vi "Base_eleve.vi"() -> ()   [LabVIEW 2018]
uses:
  <vilib>/Instr/_visa.llb/VISA Configure Serial Port (Instr).vi
panel:
  out "Array 3":dbl[](array[numeric])
  out "Array 2":dbl[](array[numeric])
  out "Array":dbl[](array[numeric])
  out "Humidity":dbl[](graph)
  out "Pressure":dbl[](graph)
  out "Temperature":dbl[](graph)
  out "Humidity":dbl
  out "Pressure":dbl
  out "Temperature":dbl
  out "Chaîne":string
  in  "stop":bool
  in  "Nom de ressource VISA":refnum<visa-resource-name>
  # "1. Brancher la carte Arduino sur un port USB\n2. Choisir le port COM de la carte dans la liste déroulante \"Nom de ressource VISA\"\n3. Lancer le programme"
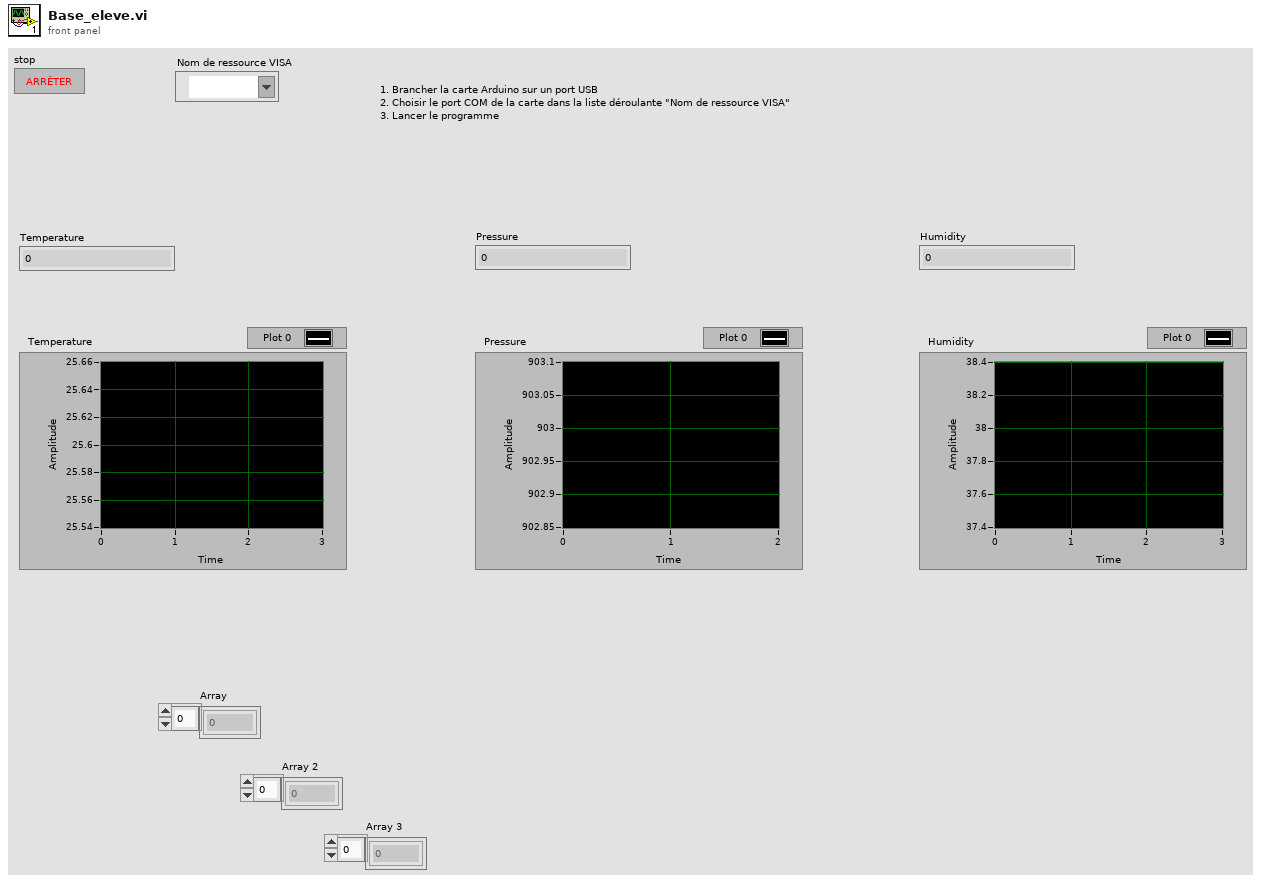
[diagram p1: front panel]
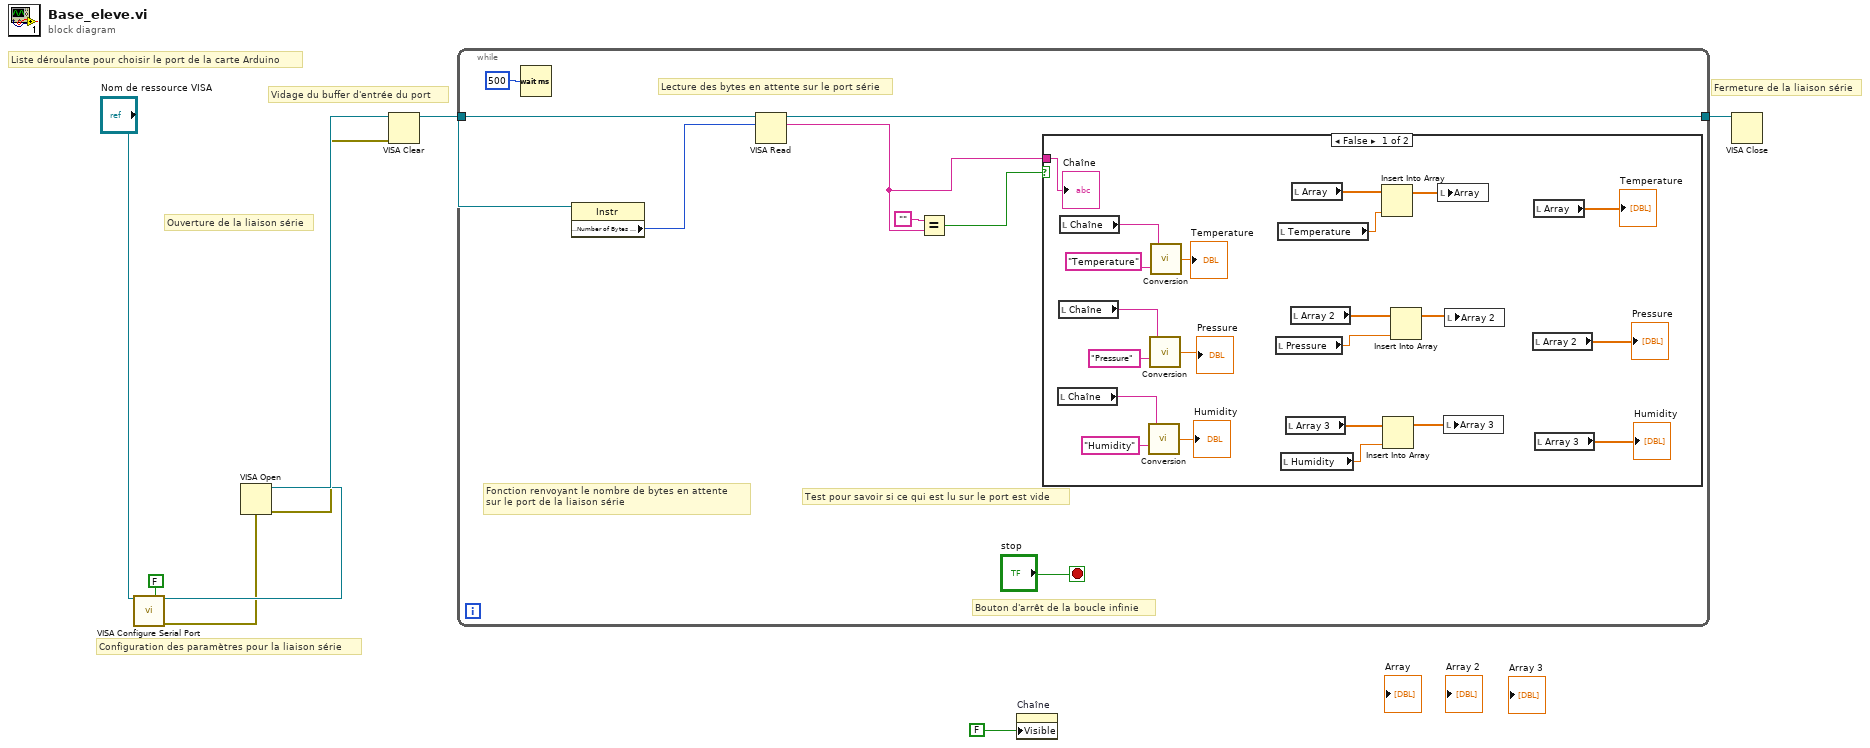
[diagram p0: block diagram]
diagram:
  # "Vidage du buffer d'entrée du port"
  # "Ouverture de la liaison série"
  # "Configuration des paramètres pour la liaison série"
  # "Liste déroulante pour choisir le port de la carte Arduino"
  # "Fermeture de la liaison série"
  n1 = call-poly "VISA Configure Serial Port"("VISA resource name"="Nom de ressource VISA", "Enable Termination\nChar (T)"=FALSE ("Enable Termination\nChar (T)")) -> ("VISA resource name out"=w6:refnum<visa-resource-name>, "error out"=w4:errorcluster)  [unwired: 12 in]
  n2 = VISA Open(error in (no error)=w4, VISA resource name=w6) -> (VISA resource name=w8:refnum<visa-resource-name>, error out=w3:errorcluster)  [unwired: 3 in]
  n3 = VISA Clear(VISA resource name=w8, error in (no error)=w3) -> (VISA resource name out=w7:refnum<visa-resource-name>)  [unwired: 1 out]
  n4 = while {
    tunnel: w7 -> [w16]
    tunnel: [w14] -> w2
    stop <- "stop" stop-if-true
    # "Lecture des bytes en attente sur le port série"
    # "Fonction renvoyant le nombre de bytes en attente\nsur le port de la liaison série"
    # "Test pour savoir si ce qui est lu sur le port est vide"
    # "Bouton d'arrêt de la boucle infinie"
    n5 = Wait (ms)(milliseconds to wait=u32 500 ("attente (ms)")) -> ()  [unwired: 1 out]
    n6 = property class="Instr"(reference=w16) -> ("Serial Settings:Number of Bytes at Serial Port"=w15:u32)  [unwired: 1 in, 2 out]
    n7 = VISA Read(VISA resource name=w16, byte count=w15) -> (VISA resource name out=w14:refnum<visa-resource-name>, read buffer=w10:string)  [unwired: 1 in, 2 out]
    n8 = Equal?(x="", y=w10) -> (x = y?=w11:bool)
    n9 = case shown="False" w11 {
      tunnel: w10 -> [w39 _]
      frame False {
        n10 = local read "Chaîne"() -> (w34:string)
        n11 = local read "Chaîne"() -> (w35:string)
        n12 = local read "Chaîne"() -> (w38:string)
        n13 = call "Conversion.vi"("String 3"="Humidity", "String"=w34) -> ("Numeric"=→"Humidity":dbl)
        n14 = call "Conversion.vi"("String 3"="Pressure", "String"=w35) -> ("Numeric"=→"Pressure":dbl)
        n15 = call "Conversion.vi"("String 3"="Temperature", "String"=w38) -> ("Numeric"=→"Temperature":dbl)
        n16 = local read "Pressure"() -> (w22:dbl)
        n17 = local read "Temperature"() -> (w28:dbl)
        n18 = local read "Humidity"() -> (w19:dbl)
        n19 = local read "Array 3"() -> (w21:dbl[])
        n20 = local read "Array 2"() -> (w25:dbl[])
        n21 = local read "Array"() -> (w29:dbl[])
        n22 = Insert Into Array(array=w29, new element=w28) -> (w27:dbl[])  [unwired: 1 in]
        n23 = Insert Into Array(array=w21, new element=w19) -> (w20:dbl[])  [unwired: 1 in]
        n24 = Insert Into Array(array=w25, new element=w22) -> (w24:dbl[])  [unwired: 1 in]
        n25 = local write "Array"(w27) -> ()
        n26 = local write "Array 3"(w20) -> ()
        n27 = local write "Array 2"(w24) -> ()
        n28 = local read "Array 2"() -> (→"Pressure":dbl[])
        n29 = local read "Array"() -> (→"Temperature":dbl[])
        n30 = local read "Array 3"() -> (→"Humidity":dbl[])
        "Chaîne" <- w39
      }
      frame True {
      }
    }
  }
  n31 = property on="Chaîne" class="Str"("Visible"=FALSE) -> ()  [unwired: 2 in, 2 out]
  n32 = VISA Close(VISA resource name=w2) -> ()  [unwired: 1 in, 1 out]
